vi "stringToXY.vi"(10 "delimiter":string, 11 "string":string) -> (2 "X":i32[](array[numeric]), 3 "Y":i32[](array[numeric]))   [LabVIEW 2023]
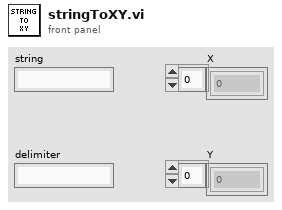
[diagram p1: front panel]
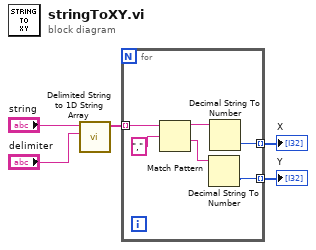
[diagram p0: block diagram]
diagram:
  n1 = call <vilib>:"Delimited String to 1D String Array.vi"("delimiter"="delimiter", "delimited string"="string") -> ("string array"=w3:string[])  [unwired: 9 in]
  n2 = for {
    tunnel: w3 -> [w11] mode=indexing
    tunnel: [w8] -> w1 mode=indexing
    tunnel: [w7] -> w2 mode=indexing
    n3 = Match Pattern(string=w11, regular expression=",") -> (before substring=w9:string, after substring=w6:string)  [unwired: 1 in, 2 out]
    n4 = Decimal String To Number(string=w6) -> (number=w7:i32)  [unwired: 2 in, 1 out]
    n5 = Decimal String To Number(string=w9) -> (number=w8:i32)  [unwired: 2 in, 1 out]
  }
  "Y" <- w2
  "X" <- w1
